vi "onTerminateSession.vi"(8 "error in (no error)":errorcluster, 10 "Destroy (T)":bool=TRUE, 11 "Session.Server in":refnum<class "Session.Server.lvclass">) -> (0 "error out":errorcluster, 2 "Session Destroyed":bool, 3 "Session.Server out":refnum<class "Session.Server.lvclass">)   [LabVIEW 2013, in "MQTT Server.lvlib" / "Session.Server.lvclass"]
uses:
  Session.Server.lvclass
  <vilib>/LabVIEW Open Source Project/MQTT Connection/MQTT_Base/Session/Session.lvclass
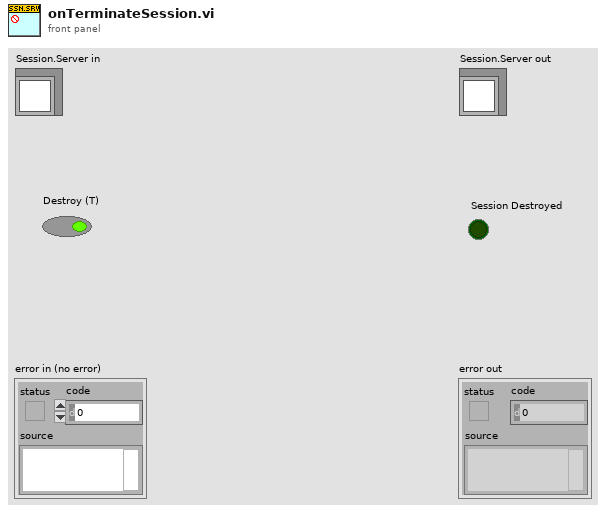
[diagram p1: front panel]
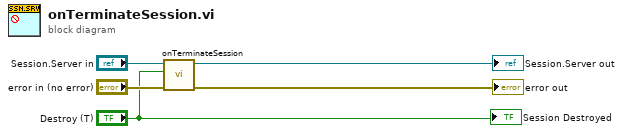
[diagram p0: block diagram]
diagram:
  n1 = call-parent "onTerminateSession.vi"("error in (no error)"="error in (no error)", "Destroy (T)"="Destroy (T)", "Session in"="Session.Server in") -> ("error out"=→"error out":errorcluster, "Session out"=→"Session.Server out":refnum<class "Session.Server.lvclass">)  [unwired: 6 in, 1 out]
  "Session Destroyed" <- "Destroy (T)"
